vi "proba_szogfugv.vi"() -> ()   [LabVIEW 2012]
panel:
  out "szögRobottoól":dbl(knob)
  out "Jobb":dbl(slide) scale=-2.0..2.0
  out "Bal":dbl(slide) scale=-2.0..2.0 scale format="%0#1_1g"
  in  "Stop Button":bool
  out "Mouse Position":cluster{"X":i32, "Y":i32}
  out "táv":dbl(slide) scale=0.0..3.0
  out "Joy":picture
  out "szögNullponttól":dbl(knob)
  out "a":dbl
  out "b":dbl
  out "y":dbl step=0.01
  out "x":dbl step=0.01
  out "XY Graph":cluster{"X":dbl[], "Y":dbl[]}[](graph)
  # "0"
  # "1,3"
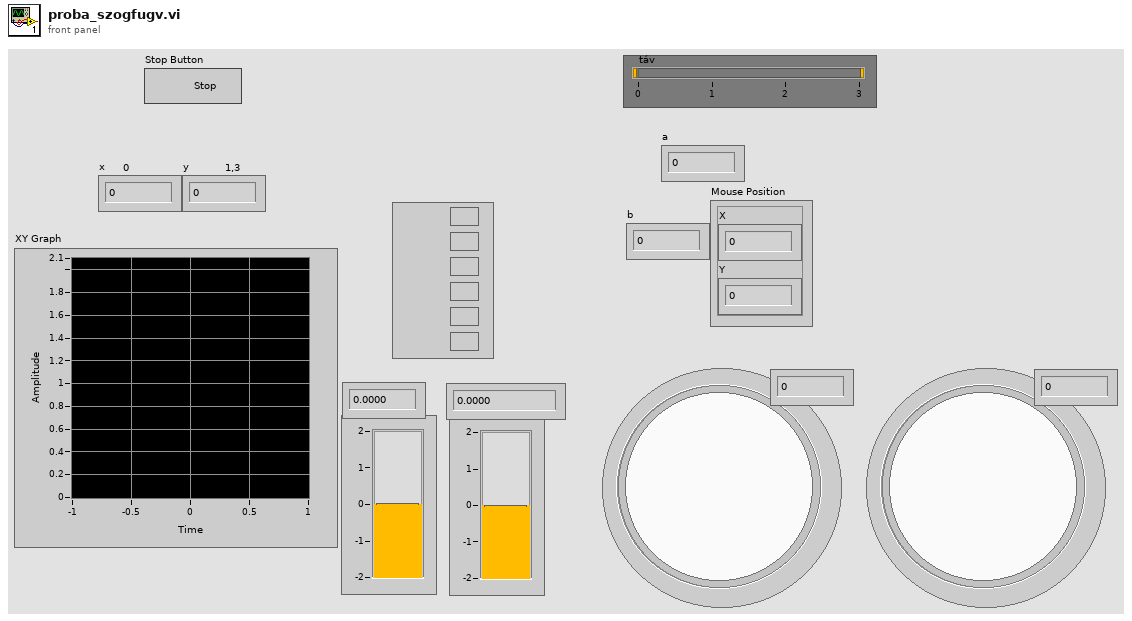
[diagram p1: front panel]
types:
  T1 = cluster{"left":i16, "top":i16, "right":i16, "bottom":i16}
  T2 = cluster{"Width":u16, "Style":enum32{"Solid", "Dash", "Dot", "DashDot", "DashDotDot"}}
  T3 = typedef "LVMouseTypeDef.ctl" = cluster{"Mouse Position":cluster{"X":i32, "Y":i32}, "Mouse Modifiers":cluster{"Button Down":bool, "Shift Mod":bool, "Menu Mod":bool, "Option Mod":bool}}
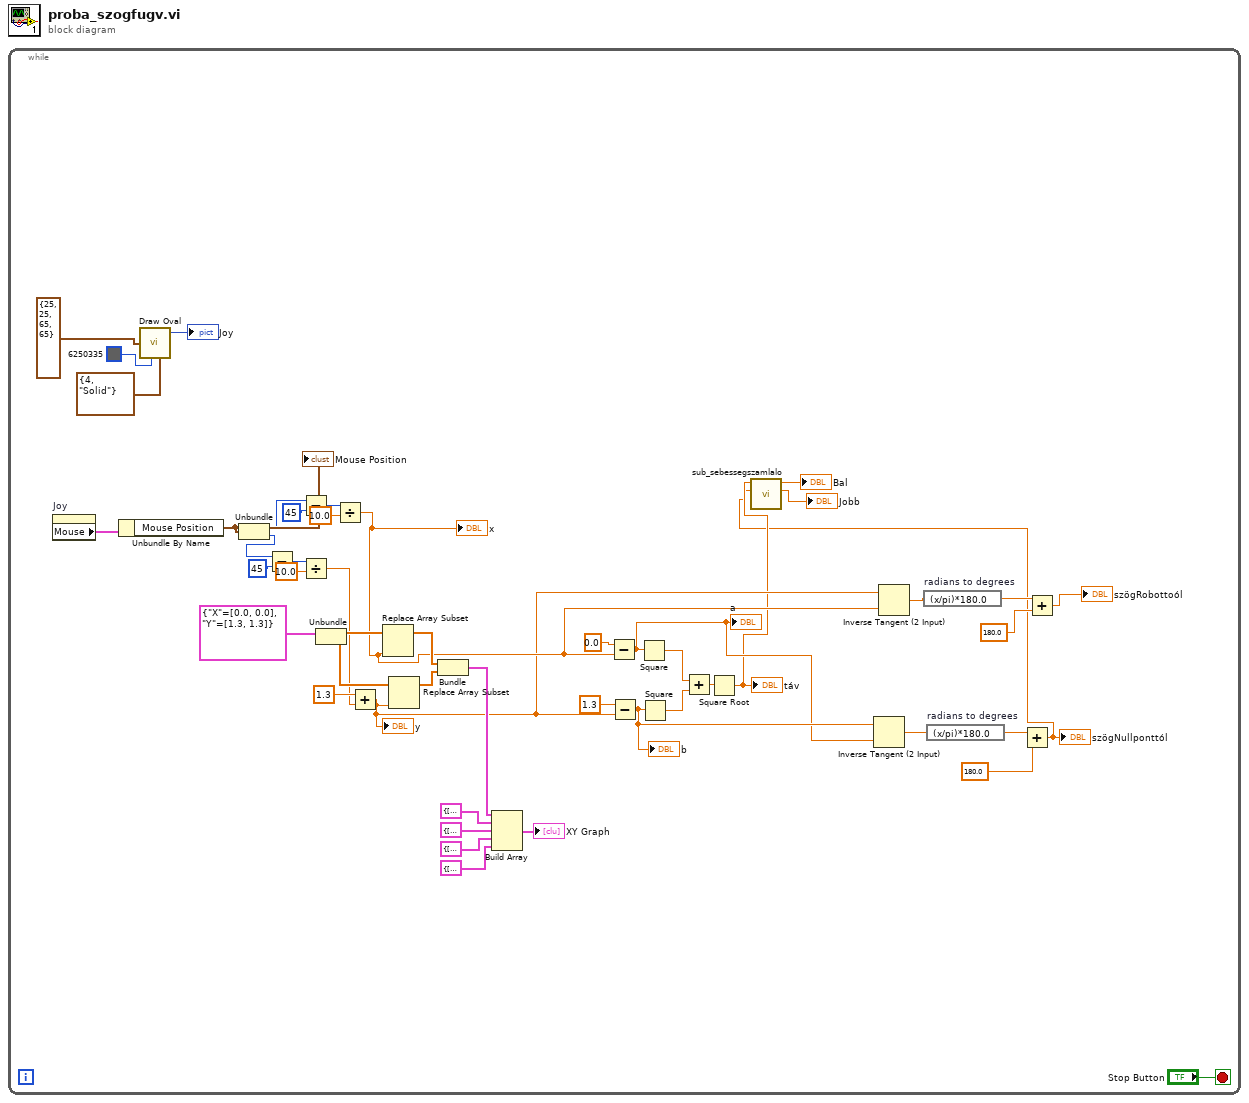
[diagram p0: block diagram]
diagram:
  n1 = while {
    stop <- "Stop Button" stop-if-true
    n2 = property on="Joy" class="Pict"() -> ("Mouse"=w30:T3)  [unwired: 2 in, 2 out]
    n3 = Unbundle By Name(w30) -> ("Mouse Position"=w29:cluster{"X":i32, "Y":i32})
    "Mouse Position" <- w29
    n4 = call <vilib>:"Draw Oval.vi"("rect"=T1 {"left"=25, "top"=25, "right"=65, "bottom"=65}, "color(black)"=u32 6250335, "pen"=T2 {"Width"=4, "Style"=enum."Solid"}) -> ("new picture"=→"Joy":picture)  [unwired: 6 in]
    n5 = Unbundle(w29) -> ("X"=w27:i32, "Y"=w20:i32)
    n6 = Subtract(x=w20, y=45) -> (x-y=w22:i32)
    n7 = Subtract(x=w27, y=45) -> (x-y=w25:i32)
    n8 = Divide(x=w22, y=10.0) -> (x/y=w13:dbl)
    n9 = Unbundle(cluster{"X":dbl[], "Y":dbl[]} {"X"=[0.0, 0.0], "Y"=[1.3, 1.3]} ("Mask")) -> ("X"=w42:dbl[], "Y"=w41:dbl[])
    n10 = Divide(x=w25, y=10.0) -> (x/y=w6:dbl)
    "x" <- w6
    n11 = Add(x=1.3 ("y"), y=w13) -> (x+y=w5:dbl)
    "y" <- w5
    n12 = Replace Array Subset(array=w42, new element=w6) -> (w40:dbl[])  [unwired: 1 in]
    n13 = Replace Array Subset(array=w41, new element=w5) -> (w39:dbl[])  [unwired: 1 in]
    n14 = Bundle("X"=w40, "Y"=w39) -> (w38:cluster{"X":dbl[], "Y":dbl[]})  [unwired: 1 in]
    n15 = Build Array(w38, cluster{"X":dbl[], "Y":dbl[]} {"X"=[0.2, 0.19753766811902757, 0.19021130325903074, 0.17820130483767357, 0.16180339887498948, 0.1414213562373095, 0.11755705045849464, 0.09079809994790937, 0.0618033988749895, 0.031286893008046185, 1.2246063538223773e-17, -0.031286893008046164, -0.06180339887498947, -0.09079809994790942, -0.11755705045849461, -0.1414213562373095, -0.16180339887498948, -0.1782013048376736, -0.1902113032590307, -0.19753766811902757, -0.2, -0.19753766811902754, -0.19021130325903074, -0.1782013048376736, -0.1618033988749895, -0.14142135623730948, -0.11755705045849452, -0.0907980999479094, -0.06180339887498952, -0.03128689300804621, -3.673819061467132e-17, 0.031286893008046136, 0.06180339887498945, 0.09079809994790948, 0.11755705045849474, 0.14142135623730948, 0.16180339887498946, 0.17820130483767363, 0.1902113032590307, 0.19753766811902754, 0.2], "Y"=[1.3, 1.3312868930080461, 1.3618033988749896, 1.3907980999479095, 1.4175570504584947, 1.4414213562373095, 1.4618033988749894, 1.4782013048376736, 1.4902113032590307, 1.4975376681190276, 1.5, 1.4975376681190276, 1.4902113032590307, 1.4782013048376736, 1.4618033988749897, 1.4414213562373095, 1.4175570504584947, 1.3907980999479093, 1.3618033988749896, 1.3312868930080461, 1.3, 1.2687131069919537, 1.2381966011250105, 1.2092019000520906, 1.1824429495415054, 1.1585786437626906, 1.1381966011250104, 1.1217986951623264, 1.1097886967409694, 1.1024623318809725, 1.1, 1.1024623318809725, 1.1097886967409694, 1.1217986951623264, 1.1381966011250106, 1.1585786437626906, 1.1824429495415054, 1.2092019000520908, 1.2381966011250105, 1.2687131069919537, 1.3]} ("Mask"), cluster{"X":dbl[], "Y":dbl[]} {"X"=[0.4, 0.39507533623805513, 0.3804226065180615, 0.35640260967534715, 0.32360679774997897, 0.282842712474619, 0.23511410091698928, 0.18159619989581874, 0.123606797749979, 0.06257378601609237, 2.4492127076447546e-17, -0.06257378601609233, -0.12360679774997894, -0.18159619989581885, -0.23511410091698923, -0.282842712474619, -0.32360679774997897, -0.3564026096753472, -0.3804226065180614, -0.39507533623805513, -0.4, -0.3950753362380551, -0.3804226065180615, -0.3564026096753472, -0.323606797749979, -0.28284271247461895, -0.23511410091698903, -0.1815961998958188, -0.12360679774997904, -0.06257378601609243, -7.347638122934264e-17, 0.06257378601609227, 0.1236067977499789, 0.18159619989581896, 0.23511410091698948, 0.28284271247461895, 0.3236067977499789, 0.35640260967534726, 0.3804226065180614, 0.3950753362380551, 0.4], "Y"=[1.3, 1.3625737860160925, 1.4236067977499791, 1.4815961998958187, 1.5351141009169893, 1.5828427124746192, 1.623606797749979, 1.6564026096753472, 1.6804226065180614, 1.6950753362380553, 1.7000000000000002, 1.6950753362380553, 1.6804226065180616, 1.656402609675347, 1.623606797749979, 1.5828427124746192, 1.5351141009169893, 1.4815961998958187, 1.4236067977499791, 1.3625737860160925, 1.3, 1.2374262139839076, 1.1763932022500212, 1.1184038001041814, 1.0648858990830108, 1.017157287525381, 0.9763932022500209, 0.9435973903246528, 0.9195773934819387, 0.904924663761945, 0.9, 0.9049246637619449, 0.9195773934819386, 0.9435973903246531, 0.9763932022500212, 1.017157287525381, 1.0648858990830108, 1.1184038001041816, 1.176393202250021, 1.2374262139839076, 1.3]} ("Mask"), cluster{"X":dbl[], "Y":dbl[]} {"X"=[0.6, 0.5926130043570826, 0.5706339097770922, 0.5346039145130207, 0.4854101966249684, 0.4242640687119285, 0.3526711513754839, 0.2723942998437281, 0.18541019662496847, 0.09386067902413855, 3.6738190614671314e-17, -0.09386067902413847, -0.1854101966249684, -0.27239429984372826, -0.3526711513754838, -0.42426406871192845, -0.4854101966249684, -0.5346039145130208, -0.570633909777092, -0.5926130043570826, -0.6, -0.5926130043570825, -0.5706339097770922, -0.5346039145130207, -0.4854101966249685, -0.4242640687119284, -0.3526711513754835, -0.27239429984372815, -0.18541019662496855, -0.09386067902413862, -1.1021457184401395e-16, 0.0938606790241384, 0.18541019662496833, 0.2723942998437284, 0.3526711513754842, 0.4242640687119284, 0.48541019662496837, 0.5346039145130209, 0.570633909777092, 0.5926130043570826, 0.6], "Y"=[1.3, 1.3938606790241386, 1.4854101966249684, 1.5723942998437281, 1.652671151375484, 1.7242640687119286, 1.7854101966249685, 1.8346039145130209, 1.870633909777092, 1.8926130043570826, 1.9, 1.8926130043570826, 1.870633909777092, 1.8346039145130206, 1.7854101966249685, 1.7242640687119286, 1.652671151375484, 1.572394299843728, 1.4854101966249686, 1.3938606790241386, 1.3, 1.2061393209758613, 1.1145898033750317, 1.027605700156272, 0.9473288486245163, 0.8757359312880715, 0.8145898033750314, 0.7653960854869793, 0.729366090222908, 0.7073869956429174, 0.7000000000000001, 0.7073869956429174, 0.7293660902229079, 0.7653960854869796, 0.8145898033750318, 0.8757359312880715, 0.947328848624516, 1.0276057001562724, 1.1145898033750314, 1.2061393209758613, 1.2999999999999998]} ("Mask"), cluster{"X":dbl[], "Y":dbl[]} {"X"=[1.0, 0.9876883405951378, 0.9510565162951535, 0.8910065241883679, 0.8090169943749475, 0.7071067811865476, 0.5877852522924731, 0.4539904997395468, 0.30901699437494745, 0.15643446504023092, 6.123031769111886e-17, -0.1564344650402308, -0.30901699437494734, -0.45399049973954714, -0.587785252292473, -0.7071067811865475, -0.8090169943749473, -0.891006524188368, -0.9510565162951535, -0.9876883405951377, -1.0, -0.9876883405951377, -0.9510565162951536, -0.8910065241883679, -0.8090169943749476, -0.7071067811865474, -0.5877852522924726, -0.4539904997395469, -0.30901699437494756, -0.15643446504023104, -1.836909530733566e-16, 0.15643446504023067, 0.30901699437494723, 0.4539904997395474, 0.5877852522924737, 0.7071067811865474, 0.8090169943749473, 0.8910065241883681, 0.9510565162951535, 0.9876883405951377, 1.0], "Y"=[1.3, 1.456434465040231, 1.6090169943749475, 1.7539904997395468, 1.8877852522924732, 2.0071067811865477, 2.1090169943749473, 2.191006524188368, 2.2510565162951535, 2.287688340595138, 2.3, 2.287688340595138, 2.2510565162951535, 2.1910065241883676, 2.1090169943749473, 2.0071067811865477, 1.8877852522924732, 1.7539904997395466, 1.6090169943749475, 1.456434465040231, 1.3000000000000003, 1.1435655349597689, 0.9909830056250528, 0.8460095002604533, 0.712214747707527, 0.5928932188134524, 0.49098300562505215, 0.40899347581163226, 0.3489434837048465, 0.3123116594048624, 0.30000000000000004, 0.3123116594048623, 0.3489434837048464, 0.4089934758116325, 0.49098300562505304, 0.5928932188134524, 0.7122147477075267, 0.8460095002604539, 0.9909830056250524, 1.1435655349597689, 1.2999999999999998]} ("Mask")) -> (→"XY Graph":cluster{"X":dbl[], "Y":dbl[]}[])
    n16 = Subtract(x=0.0, y=w6) -> (x-y=w7:dbl)
    "a" <- w7
    n17 = Subtract(x=1.3 ("y"), y=w5) -> (x-y=w12:dbl)
    "b" <- w12
    n18 = Square(x=w7) -> (x^2=w35:dbl)
    n19 = Square(x=w12) -> (x^2=w34:dbl)
    n20 = Add(x=w35, y=w34) -> (x+y=w19:dbl)
    n21 = Square Root(x=w19) -> (sqrt(x)=w4:dbl)
    "táv" <- w4
    n22 = Inverse Tangent (2 Input)(1:w7, 2:w12) -> (0:w33:dbl)
    n23 = Inverse Tangent (2 Input)(1:w6, 2:w5) -> (0:w11:dbl)
    n24 = expression code="(x/pi)*180.0" "radians to degrees"(w11) -> (w10:dbl)
    n25 = expression code="(x/pi)*180.0" "radians to degrees"(w33) -> (w32:dbl)
    n26 = Add(x=w32, y=180.0) -> (x+y=w3:dbl)
    "szögNullponttól" <- w3
    n27 = call "sub_sebessegszamlalo.vi"("Szög"=w3, "Táv"=w4) -> ("Jobb"=→"Jobb":dbl, "Bal"=→"Bal":dbl)  [unwired: 8 in]
    n28 = Add(x=w10, y=180.0) -> (x+y=→"szögRobottoól":dbl)
  }
